vi "Table Stage Manufacturer Model - FGV.vi"(7 "Actions":T1=enum."Clear", 8 "Error In":errorcluster, 11 "Stage MFG/Model [In]":cluster{"X":T2, "Y":T2, "Z":T2}) -> (0 "Error Out":errorcluster, 3 "Stage MFG/Model [Out]":cluster{"X":T2, "Y":T2, "Z":T2})   [LabVIEW 2014]
uses:
  General/Controls/Translation Stage Types.ctl
  General/Controls/FGV Actions.ctl
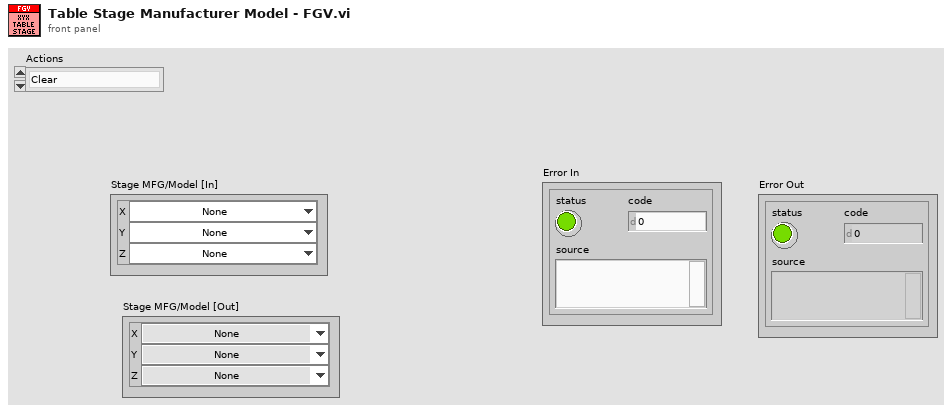
[diagram p1: front panel]
types:
  T1 = typedef "FGV Actions.ctl" = enum16{"Init", "Set", "Get", "Clear"}
  T2 = typedef "Translation Stage Types.ctl" = enum16{"None", "Thorlabs LTS", "Thorlabs MLJ"}
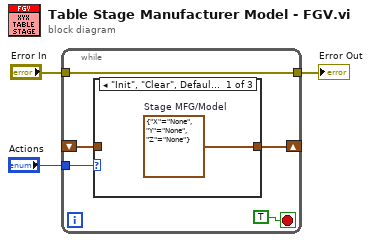
[diagram p0: block diagram]
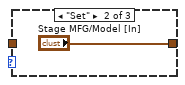
[diagram p2: hidden frame]
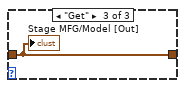
[diagram p3: hidden frame]
diagram:
  n1 = while {
    tunnel: "Actions" -> [w8]
    shift-right: [w6] -> _
    shift-left: _ -> [w5]
    tunnel: [w4] -> w2
    tunnel: "Error In" -> [w4]
    stop <- TRUE stop-if-true
    n2 = case shown="\"Init\", \"Clear\", Default" w8 {
      tunnel: [w9 "Stage MFG/Model [In]" w11] -> w6
      tunnel: w5 -> [_ _ w11]
      frame "Init", "Clear", Default {
        w9 = cluster{"X":T2, "Y":T2, "Z":T2} {"X"=enum."None", "Y"=enum."None", "Z"=enum."None"}  # Stage MFG/Model
      }
      frame "Set" {
      }
      frame "Get" {
        "Stage MFG/Model [Out]" <- w11
      }
    }
  }
  "Error Out" <- w2
